vi "BuildServerTitleText.vi"(3 "ROS":T1={"topic port"=0, "Node"="", "topic"="", "type"="", "node port"=0, "error "={"status"=FALSE, "code"=0, "source"=""}, "Direction"=enum."Node", "Update (ms)"=1, "queue size"=0}) -> (0 "text":string, 1 "colored text":string)   [LabVIEW 2012]
doc: "Builds server title for website logs"
uses:
  <userlib>/ROSforLV/ROS/Code/SubVIs/_ROSControl.ctl
  <userlib>/ROSforLV/ROS/Code/SubVIs/_ROSDirection.ctl
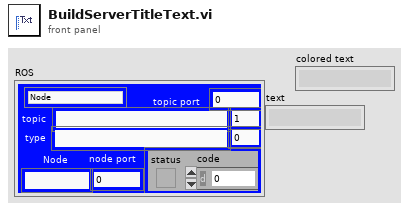
[diagram p1: front panel]
types:
  T1 = typedef "_ROSControl.ctl" = cluster{"topic port":u16, "Node":string, "topic":string, "type":string, "node port":u16, "error ":errorcluster, "Direction":T2, "Update (ms)":u16, "queue size":u16}
  T2 = typedef "_ROSDirection.ctl" = enum16{"Node", "Publisher", "Subscriber", "Service Client"}
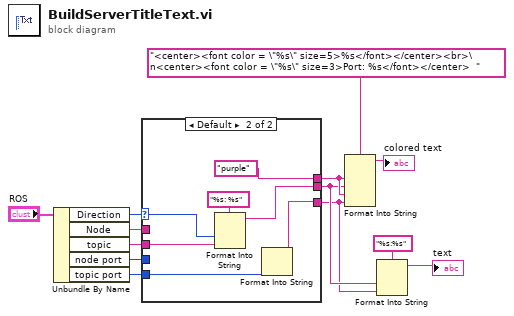
[diagram p0: block diagram]
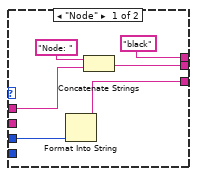
[diagram p2: hidden frame]
diagram:
  n1 = Unbundle By Name("ROS") -> ("Direction"=w10:T2, "Node"=w11:string, "topic"=w12:string, "node port"=w6:u16, "topic port"=w5:u16)
  n2 = case shown="Default" w10 {
    selector: w10 -> [_ w25]
    tunnel: w11 -> [w17 _]
    tunnel: w12 -> [_ w24]
    tunnel: [w16 w23] -> w3
    tunnel: ["black" ("format string") "purple" ("format string")] -> w7
    tunnel: w6 -> [w15 _]
    tunnel: [w14 w20] -> w2
    tunnel: w5 -> [_ w21]
    frame "Node" {
      n3 = Format Into String(w15) -> (resulting string=w14:string)  [unwired: 3 in, 1 out]
      n4 = Concatenate Strings("Node: " ("format string"), w17) -> (w16:string)
    }
    frame Default {
      n5 = Format Into String(format string="%s: %s", w25, w24) -> (resulting string=w23:string)  [unwired: 2 in, 1 out]
      n6 = Format Into String(w21) -> (resulting string=w20:string)  [unwired: 3 in, 1 out]
    }
  }
  n7 = Format Into String(format string="<center><font color = \"%s\" size=5>%s</font></center><br>\n<center><font color = \"%s\" size=3>Port: %s</font></center>  " ("string"), w7, w3, w7, w2) -> (resulting string=→"colored text":string)  [unwired: 2 in, 1 out]
  n8 = Format Into String(format string="%s:%s", w3, w2) -> (resulting string=→"text":string)  [unwired: 2 in, 1 out]
